vi "launch process event pair bag.vi"(6 "launch items":T1, 7 "bag action":T3, 11 "even pair IN":T2) -> (1 "Keys":T1[](array[typedef]), 3 "even pair OUT":T2)   [LabVIEW 2020]
uses:
  launch items list.ctl
  que event bag action.ctl
  server talk-to-back pair.ctl
  server talkback message type.ctl
  server talkto message type.ctl
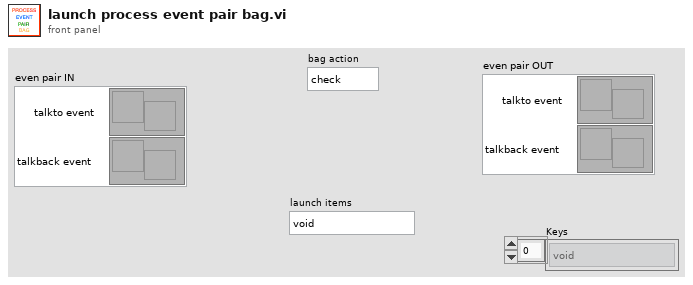
[diagram p1: front panel]
types:
  T1 = typedef "launch items list.ctl" = enum16{"void", "source", "pll engine", "pll monitor", "sweeper engine", "sweeper monitor", "fitter", "--Keys"}
  T2 = typedef "server talk-to-back pair.ctl" = cluster{"talkback event":refnum<user-event>, "talkto event":refnum<user-event>}
  T3 = typedef "que event bag action.ctl" = enum16{"check", "add", "init"}
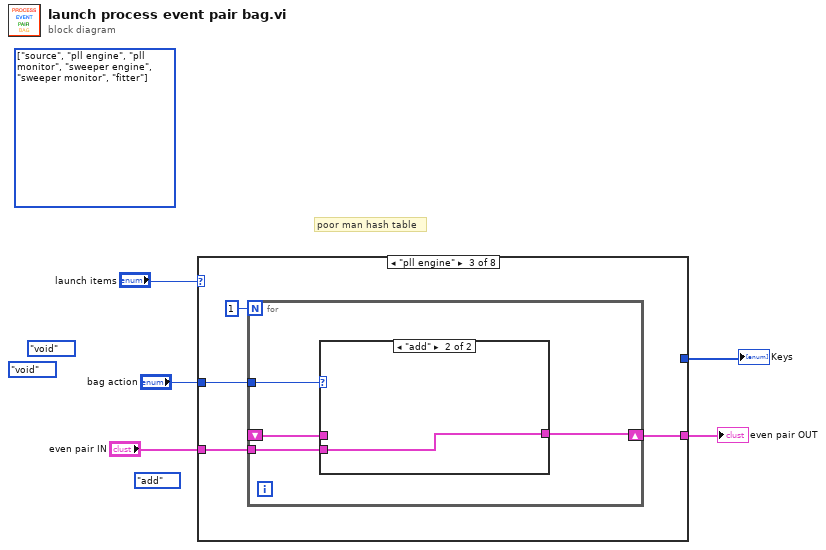
[diagram p0: block diagram]
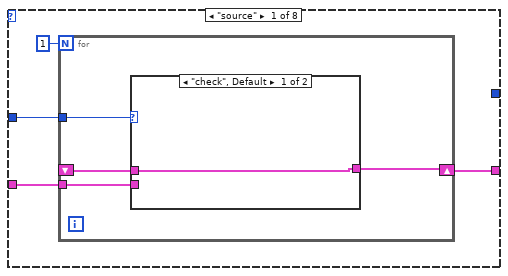
[diagram p2: hidden frame]
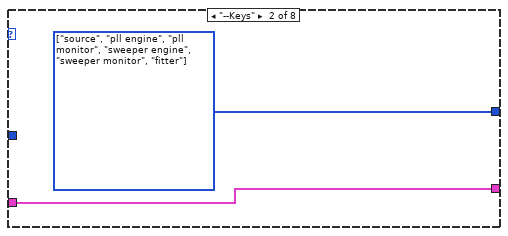
[diagram p4: hidden frame]
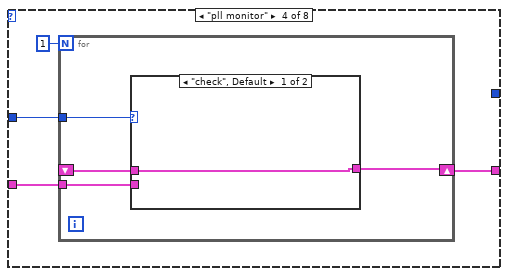
[diagram p6: hidden frame]
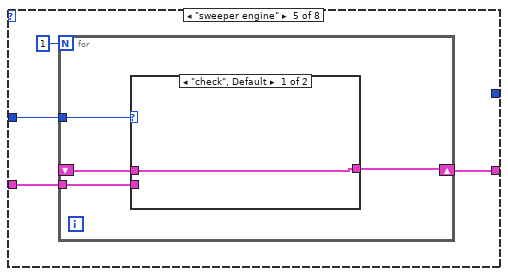
[diagram p8: hidden frame]
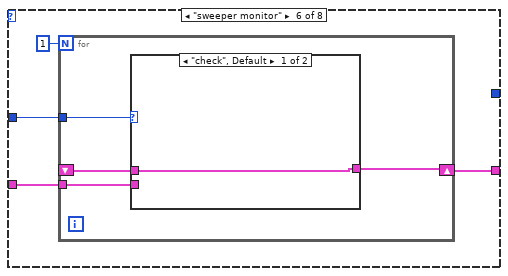
[diagram p10: hidden frame]
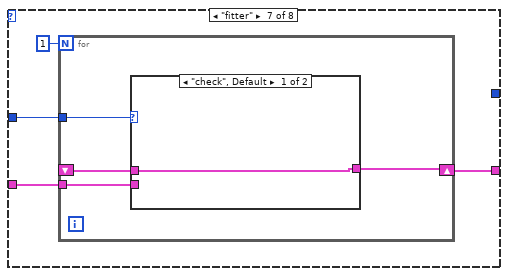
[diagram p12: hidden frame]
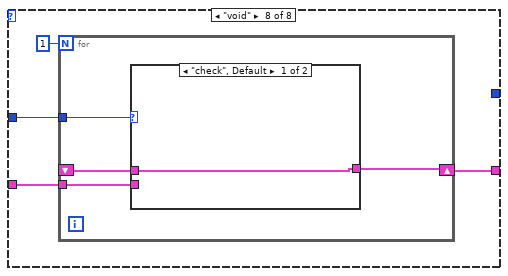
[diagram p14: hidden frame]
diagram:
  (unwired) T1[] [enum."source", enum."pll engine", enum."pll monitor", enum."sweeper engine", enum."sweeper monitor", enum."fitter"] items=["void", "source", "pll engine", "pll monitor", "sweeper engine", "sweeper monitor", "fitter", "--Keys"]
  (unwired) launch_items_list."void" ("launch items")
  (unwired) launch_items_list."void" ("launch items")
  (unwired) que_event_bag_action."add" ("bag action")
  # "poor man hash table"
  n1 = case shown="\"pll engine\"" "launch items" {
    tunnel: "even pair IN" -> [w8 w17 w20 w30 w40 w50 w60 w70]
    tunnel: "bag action" -> [w7 _ w19 w29 w39 w49 w59 w69]
    tunnel: [w6 w17 w18 w28 w38 w48 w58 w68] -> w3
    tunnel: [_ w16 _ _ _ _ _ _] -> w1
    frame "source" {
      n2 = for {
        N: 1 -> [_]
        tunnel: w8 -> [w11]
        tunnel: w7 -> [w13]
        shift-right: [w12] -> w6
        shift-left: _ -> [w10]
        n3 = case shown="\"check\", Default" w13 {
          tunnel: [w14 w15] -> w12
          tunnel: w11 -> [_ w15]
          tunnel: w10 -> [w14 _]
          frame "check", Default {
          }
          frame "add" {
          }
        }
      }
    }
    frame "--Keys" {
      w16 = T1[] [enum."source", enum."pll engine", enum."pll monitor", enum."sweeper engine", enum."sweeper monitor", enum."fitter"] items=["void", "source", "pll engine", "pll monitor", "sweeper engine", "sweeper monitor", "fitter", "--Keys"]
    }
    frame "pll engine" {
      n4 = for {
        N: 1 -> [_]
        tunnel: w20 -> [w23]
        tunnel: w19 -> [w25]
        shift-right: [w24] -> w18
        shift-left: _ -> [w22]
        n5 = case shown="\"add\"" w25 {
          tunnel: [w26 w27] -> w24
          tunnel: w23 -> [_ w27]
          tunnel: w22 -> [w26 _]
          frame "check", Default {
          }
          frame "add" {
          }
        }
      }
    }
    frame "pll monitor" {
      n6 = for {
        N: 1 -> [_]
        tunnel: w30 -> [w33]
        tunnel: w29 -> [w35]
        shift-right: [w34] -> w28
        shift-left: _ -> [w32]
        n7 = case shown="\"check\", Default" w35 {
          tunnel: [w36 w37] -> w34
          tunnel: w33 -> [_ w37]
          tunnel: w32 -> [w36 _]
          frame "check", Default {
          }
          frame "add" {
          }
        }
      }
    }
    frame "sweeper engine" {
      n8 = for {
        N: 1 -> [_]
        tunnel: w40 -> [w43]
        tunnel: w39 -> [w45]
        shift-right: [w44] -> w38
        shift-left: _ -> [w42]
        n9 = case shown="\"check\", Default" w45 {
          tunnel: [w46 w47] -> w44
          tunnel: w43 -> [_ w47]
          tunnel: w42 -> [w46 _]
          frame "check", Default {
          }
          frame "add" {
          }
        }
      }
    }
    frame "sweeper monitor" {
      n10 = for {
        N: 1 -> [_]
        tunnel: w50 -> [w53]
        tunnel: w49 -> [w55]
        shift-right: [w54] -> w48
        shift-left: _ -> [w52]
        n11 = case shown="\"check\", Default" w55 {
          tunnel: [w56 w57] -> w54
          tunnel: w53 -> [_ w57]
          tunnel: w52 -> [w56 _]
          frame "check", Default {
          }
          frame "add" {
          }
        }
      }
    }
    frame "fitter" {
      n12 = for {
        N: 1 -> [_]
        tunnel: w60 -> [w63]
        tunnel: w59 -> [w65]
        shift-right: [w64] -> w58
        shift-left: _ -> [w62]
        n13 = case shown="\"check\", Default" w65 {
          tunnel: [w66 w67] -> w64
          tunnel: w63 -> [_ w67]
          tunnel: w62 -> [w66 _]
          frame "check", Default {
          }
          frame "add" {
          }
        }
      }
    }
    frame "void" {
      n14 = for {
        N: 1 -> [_]
        tunnel: w70 -> [w73]
        tunnel: w69 -> [w75]
        shift-right: [w74] -> w68
        shift-left: _ -> [w72]
        n15 = case shown="\"check\", Default" w75 {
          tunnel: [w76 w77] -> w74
          tunnel: w73 -> [_ w77]
          tunnel: w72 -> [w76 _]
          frame "check", Default {
          }
          frame "add" {
          }
        }
      }
    }
  }
  "even pair OUT" <- w3
  "Keys" <- w1
